vi "LIDAR 5.1 Unified Version V1.vi"() -> ()   [LabVIEW 2015]
uses:
  Controls/FPGA Nain State.ctl
  Controls/AI Slave State.ctl
  <vilib>/Platform/TimedLoop/XDataNode/timing_clust.ctl
  <vilib>/Platform/TimedLoop/XDataNode/nitl_modes.ctl
  <vilib>/Platform/TimedLoop/XDataNode/wakeup.ctl
  <vilib>/rvi/Emulation/niFpgaGetClockAttributes.vi
  <vilib>/rvi/Emulation/niFpgaSctlEmulationGetInTimedLoop.vi
  <vilib>/rvi/Emulation/niFpgaEmulationReportErrorSimple.vi
  <vilib>/rvi/eio/common/nirviEmuTemplateMethod_errors.vi
  <vilib>/rvi/Emulation/niFpgaCriticalErrorInLSC.vi
  LIDAR Slave Globals.vi
  <vilib>/rvi/Emulation/niFpgaProcessEmulError.vi
  <vilib>/rvi/Memory/Memory_Emulation/nirvimemoryFastEmulation.vi
  <vilib>/rvi/Memory/Memory_Emulation/nirvimemoryEmulation.vi
  <vilib>/rvi/Emulation/niFpgaEmulationIsFPGAContextNoSignature.vi
  <vilib>/rvi/DataTransferAndStorage/Container/Common/niFpgaContainerGetUniqueNameForEmu.vi
  <vilib>/rvi/errors/nirviReportUnexpectedCaseInternalError (U32).vi
  <vilib>/rvi/errors/niFpgaSetErrorForExecOnDevCompSimple.vi
  <vilib>/rvi/eio/common/nirviEmuReportErrorAndStop.vi
  <vilib>/rvi/FIFO/Fifo_Resource/nirvififoEmulationSetSize.vi
  <vilib>/rvi/FIFO/Fifo_Resource/nirviFifoEmulationQueueMgr.vi
  <instcachedir>/0/nirviFifoEmulationQueueMgr_E5CAEC123FF24DC58D834DCA3CDAA9B5.lvgen/nirviFifoEmulationQueueMgr_E5CAEC123FF24DC58D834DCA3CDAA9B5_003.vi
  <vilib>/Utility/error.llb/Clear Errors.vi
  <vilib>/rvi/FIFO/Fifo_Resource/nirvififoEmulationCreateLock.vi
  <vilib>/rvi/FIFO/Fifo_Resource/nirvififoEmulationObtainLock.vi
  <vilib>/rvi/FIFO/Fifo_Resource/nirvififoEmulationReleaseLock.vi
  <vilib>/rvi/occurrence/nirviWaitOnOccurrenceBase.vi
  <vilib>/rvi/errors/nirviReportUnexpectedCaseInternalError.vi
  <instcachedir>/0/nirviFifoEmulationQueueMgr_E5CAEC123FF24DC58D834DCA3CDAA9B5.lvgen/nirviFifoEmulationQueueMgr_E5CAEC123FF24DC58D834DCA3CDAA9B5_001.vi
  <vilib>/rvi/FIFO/Fifo_Resource/nirvififoEmulationDetermineInputValidOut.vi
  <vilib>/rvi/interface/RandomDataEmulation/niFpgaRandomDataHandleErrors.vi
  <vilib>/eio/EIONode/EIONode.xnode
  <vilib>/Platform/TimedLoop/XDataNode/XDataNode.xnode
  <vilib>/rvi/DataTransferAndStorage/Container/XNode/niFpgaContainer.xnode
  <vilib>/rvi/FIFO/Fifo_Resource/nirvififoEmulationRead.vi
  <vilib>/eio/EIOMethodNode/EIOMethodNode.xnode
  <vilib>/rvi/FIFO/Fifo_Resource/nirvififoEmulationWrite.vi
  <vilib>/rvi/interface/RandomDataEmulation/nirviRandomDataFpgaReadWriteTemplate.vi
  <vilib>/Platform/TimedLoop/XDataNode/XDNodeRunTimeDep.lvlib
  LIDAR V2 Globals.vi
panel:
  in  "Mode":bool
  in  "ResetTimeout":bool
  out "DMATimeout":bool
  in  "DebugValues":bool
  in  "TrigTimeout":u32=10000
  in  "OverrideTrig":bool
  out "SimSensID":u8
  out "FirstIterration":bool
  out "SamplesAmpount":u8
  out "VCSL#":u8
  out "AI Slave State":T1=enum."Error"
  in  "WriteSensAdd":i16
  in  "WriteSenseData":i16
  in  "WriteSensDataEn":bool
  out "User Command Idle":bool
  out "User Command Status":u8
  out "User Error":bool
  out "Configured?":bool
  out "PLL Locked":bool
  in  "User Data 0":u8
  in  "User Data 1":u8
  in  "User Command":u8
  in  "User Command Commit":bool
  in  "VgaAdd":u32
  in  "VgaData":i16
  in  "FillVga":bool
  in  "PowerBit0":bool
  in  "PowerBit1":bool
  in  "ActiveLedIndexDeb":u16
  in  "LedScanDebEn":bool
  out "Port0":u8=2 format="%.0b"
  out "Port1Bit4":bool
  out "Port1Bit5":bool
  out "Port1":u8 format="%.0b"
  in  "ScanMode":bool
  out "PulseIndex":i16=88
  in  "StartAcq":u16=26
  in  "StartPulse":u16=20
  in  "StartES":u16=15
  in  "StopES":u16=30
  out "EnableSignal":bool
  in  "PulseEnd":u16=25
  in  "DOActivate":u16=10
  in  "SendAiCMD":u16
  in  "NoOfSamples":u16=1247
  in  "AiNoOfSamples":u16
  in  "SensorMap":u8[](array[numeric])=[0, 0, 0, 0, 0, 0, 0, 0, 0, 0, 0, 0, 1, 1, 1, 1, 1, 1, 1, 1, 1, 1, 1, 1, 0, 0, 0, 0, 0, 0, 0, 0, 0, 0, 0, 0, 1, 1, 1, 1, 1, 1, 1, 1, 1, 1, 1, 1, 2, 2, 2, 2, 2, 2, 2, 2, 2, 2, 2, 2, 3, 3, 3, 3, 3, 3, 3, 3, 3, 3, 3, 3, 2, 2, 2, 2, 2, 2, 2, 2, 2, 2, 2, 2, 3, 3, 3, 3, 3, 3, 3, 3, 3, 3, 3, 3]
  in  "ActiveSensDeb":u8
  in  "SensScanDeb":bool
  in  "SendDebugVal":bool
  in  "EndOfPulseGen":bool=TRUE
  in  "SamplingEnable":bool
  in  "SingleFrame":bool
  out "MainState":T2=enum."ActivatePulseCycle"
  in  "NoOfLeds":u16=95
  in  "PulsePerLed":i16=199
  out "ActiveLedIndex":u16=2
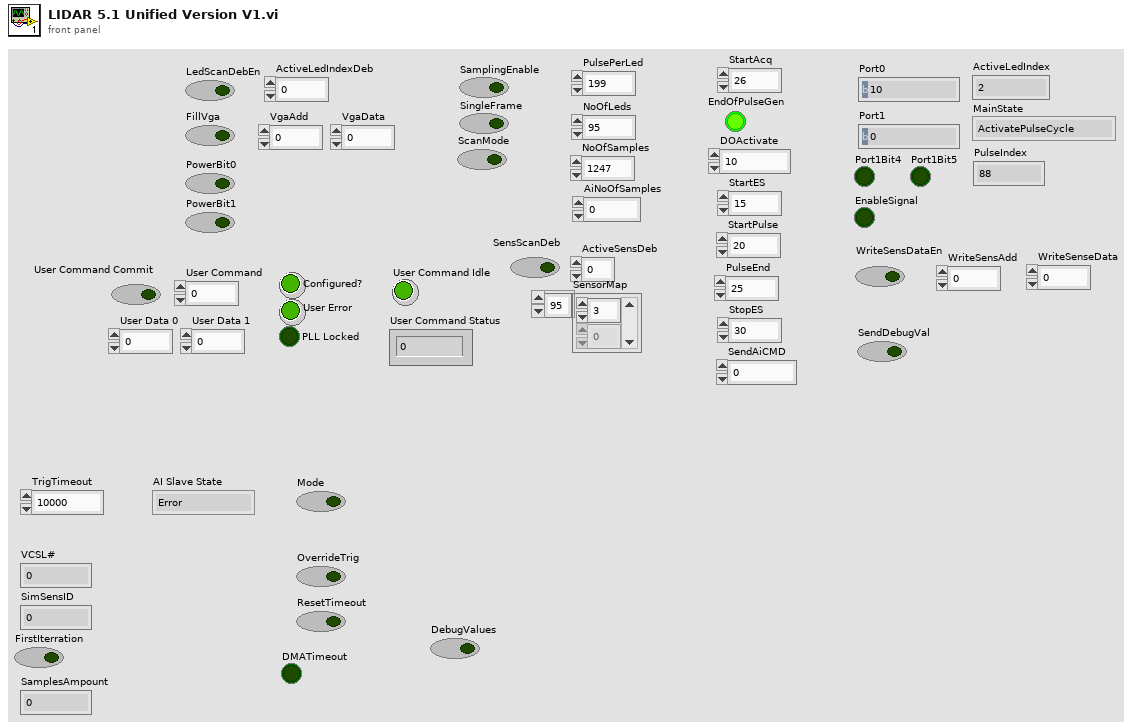
[diagram p1: front panel]
types:
  T1 = typedef "AI Slave State.ctl" = enum8{"WaitForStart", "WaitForTrig", "Read AI", "Error"}
  T2 = typedef "FPGA Nain State.ctl" = enum16{"WaitForStart", "SelectActiveLed", "WaitForNextPulse", "ActivatePulseCycle", "Error"}
  T3 = typedef "XDNodeRunTimeDep.lvlib/timing_clust.ctl" = cluster{"Expected End [f-1]":u64, "Actual End [f-1]":u64, "Finished Late? [f-1]":bool, "Expected End [i-1]":u64, "Actual End [i-1]":u64, "Finished Late? [i-1]":bool, "Expected Start [i]":u64, "Actual Start [i]":u64, "Expected Start [f]":u64, "Actual Start [f]":u64, "Source Name":string, "Structure Name":string, "Period":i64, "Deadline":i64, "Offset":i64, "Start":i64, "Priority":i32, "Timeout":i32, "Mode":T4, "Wakeup Reason":T5, "Error":errorcluster, "Source Type":string, "Secondary Source Type":string, "Global End Time":u64, "Global Start Time":u64, "Frame Duration":u64, "Iteration Duration":u64, "Assigned CPU":i32, "I/O Scan Engine Mode":u32}
  T4 = typedef "XDNodeRunTimeDep.lvlib/nitl_modes.ctl" = enum32{"No Change", "Process missed periods, maintain original phase", "Discard missed periods, maintain original phase", "Process missed periods, ignore original phase", "Discard missed periods, ignore original phase"}
  T5 = typedef "XDNodeRunTimeDep.lvlib/wakeup.ctl" = enum32{"Normal", "Aborted", "Asynchronous wakeup", "Timing source error", "Timed loop error", "Timeout"}
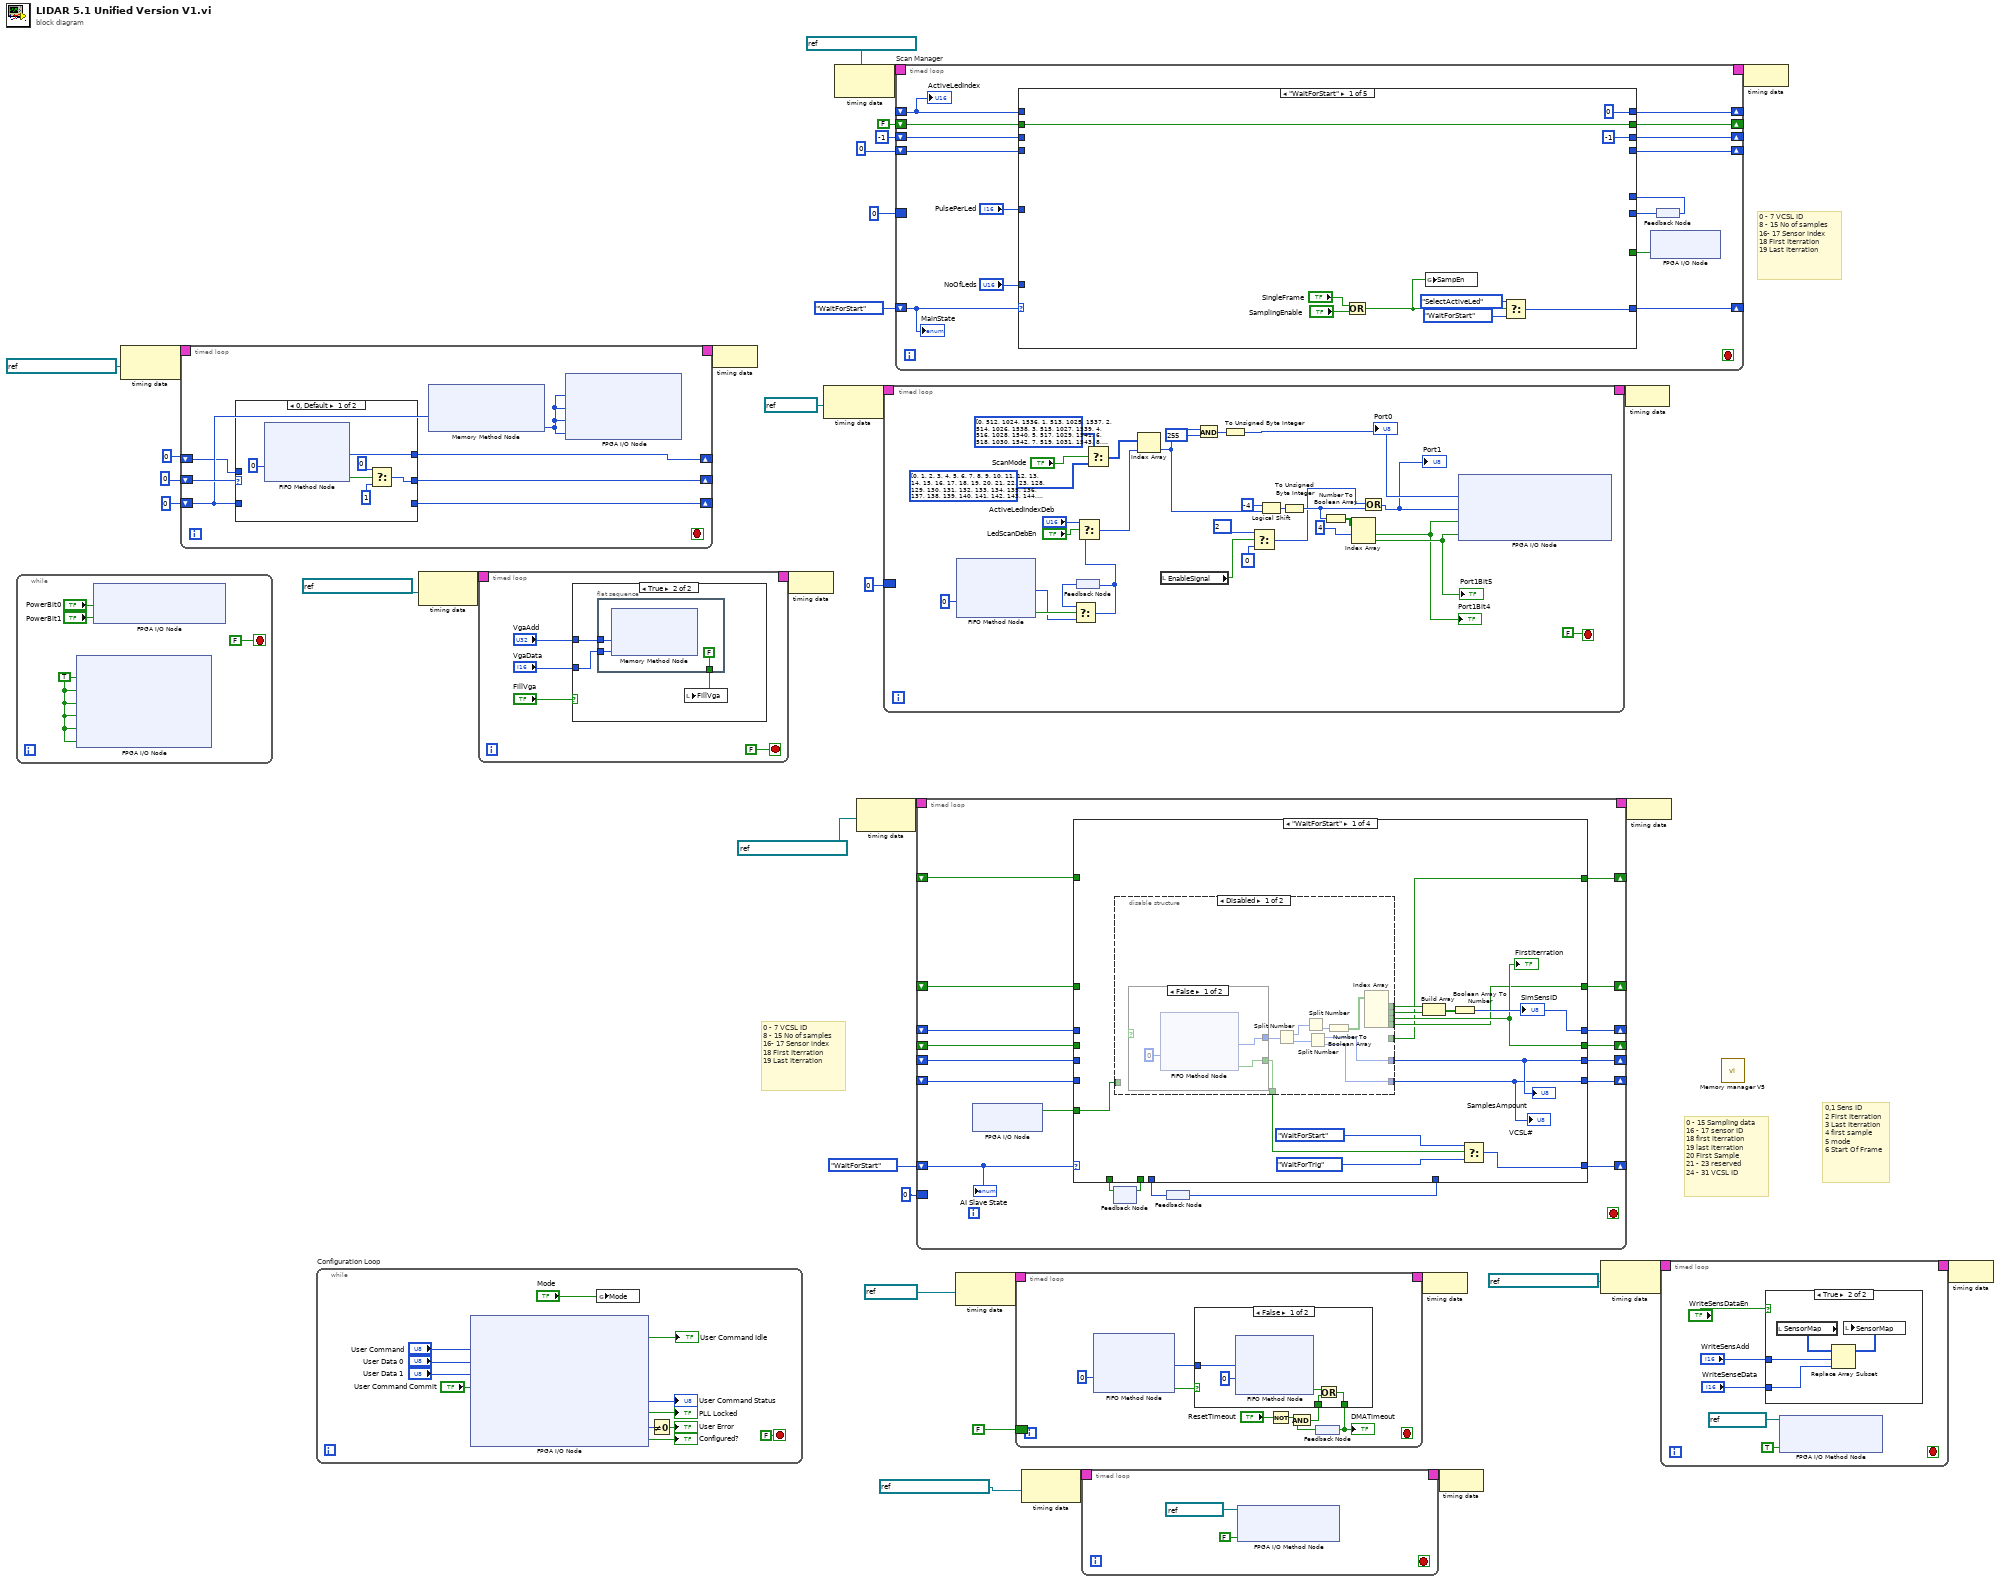
[diagram p0: block diagram]
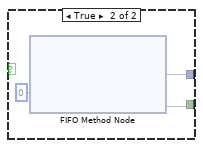
[diagram p3: hidden frame]
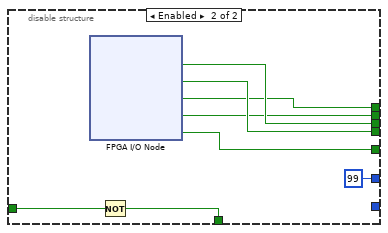
[diagram p4: hidden frame]
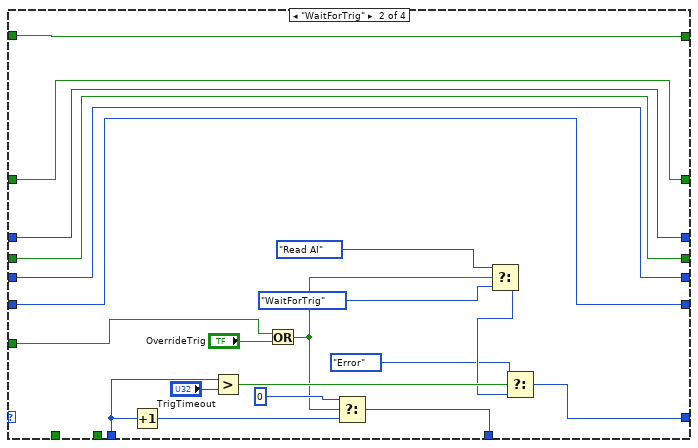
[diagram p5: hidden frame]
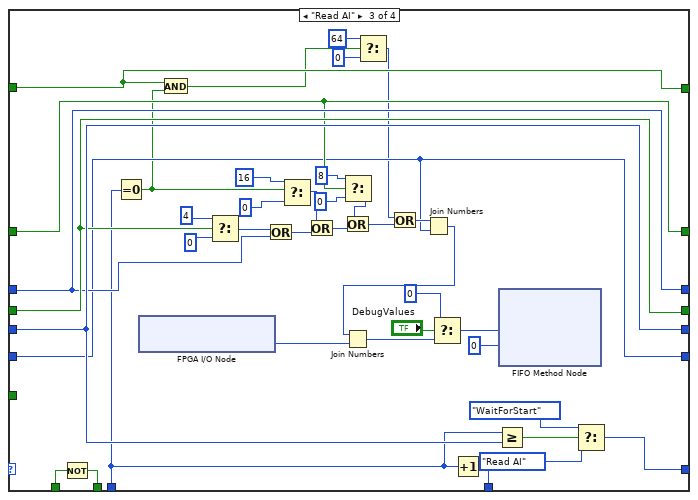
[diagram p6: hidden frame]
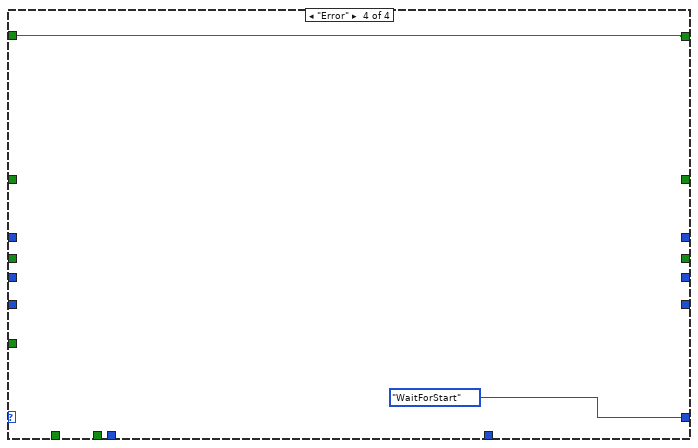
[diagram p7: hidden frame]
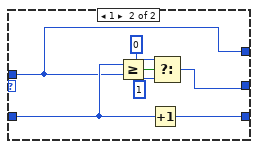
[diagram p9: hidden frame]
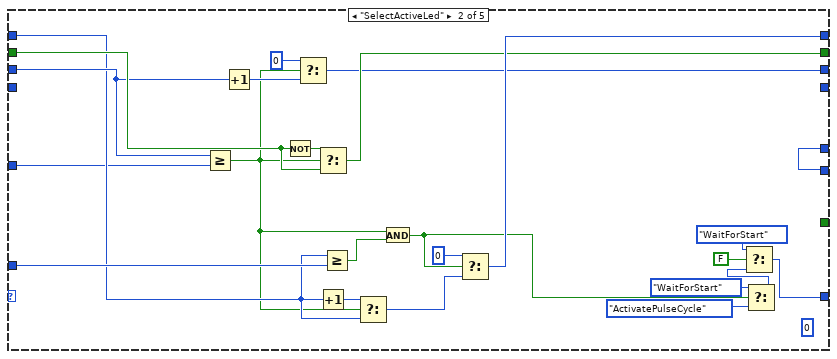
[diagram p11: hidden frame]
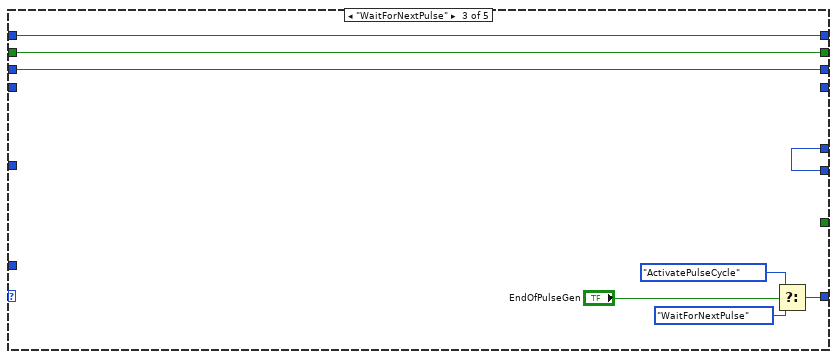
[diagram p12: hidden frame]
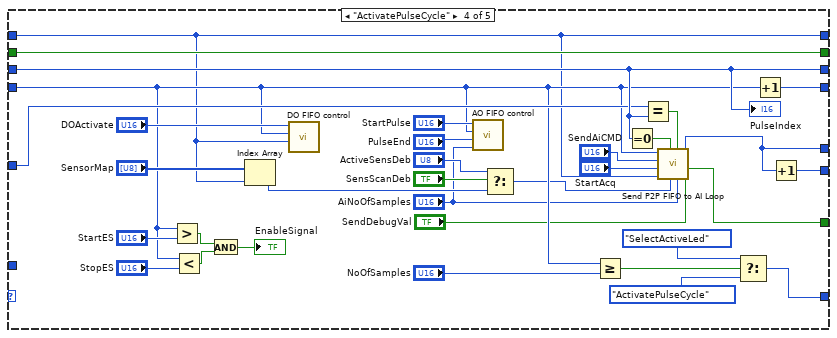
[diagram p13: hidden frame]
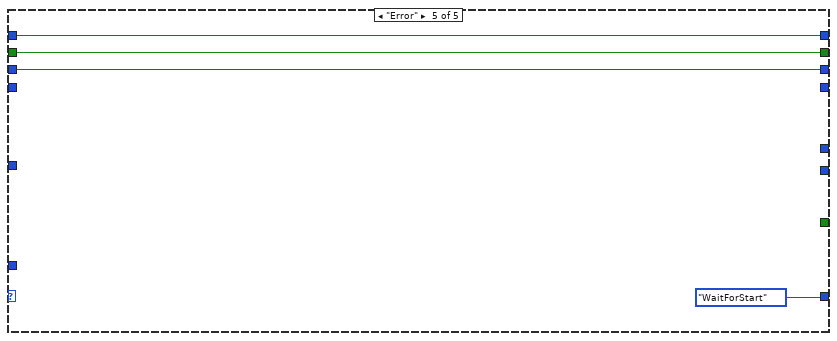
[diagram p14: hidden frame]
diagram:
  # "0,1 Sens ID\n2 First Iterration\n3 Last Iterration\n4 first sample\n5 mode\n6 Start Of Frame"
  # "0 - 15 Sampling data\n16 - 17 sensor ID\n18 first iterration\n19 last iterration\n20 First Sample\n21 - 23 reserved\n24 - 31 VCSL ID"
  # "0 - 7 VCSL ID\n8 - 15 No of samples\n16- 17 Sensor index\n18 First Iterration\n19 Last Iterration"
  # "0 - 7 VCSL ID\n8 - 15 No of samples\n16- 17 Sensor index\n18 First Iterration\n19 Last Iterration"
  n1 = while {
    stop <- FALSE stop-if-true
    w37 = TRUE ("IO Module\\PFI 0 WE")
    n2 = xnode "FPGA I/O Node"("IO Module\\PFI 0 WE"=w37, "IO Module\\PFI 1 WE"=w37, "IO Module\\PFI 2 WE"=w37, "IO Module\\PFI 3 WE"=w37, "IO Module\\DIO Port 0 WE"=w37, "IO Module\\DIO Port 1 WE"=w37) -> ()  [unwired: 6 in, 6 out]
    n3 = xnode "FPGA I/O Node"("IO Module\\PFI 2 Wr Data"="PowerBit0", "IO Module\\PFI 3 Wr Data"="PowerBit1") -> ()  [unwired: 2 in, 2 out]
  }
  n4 = node-c288(refnum<k21> "IO Module\\Data Clock" ("Source Name")) -> (w30:T3)
  n5 = timed-loop {
    timing: w30 -> [_]
    timing-out: [_] -> w29
    shift-right: [w44] -> _
    shift-left: u16 0 -> [w43]
    shift-right: [w45] -> _
    shift-left: u8 0 -> [w46]
    shift-right: [w42] -> _
    shift-left: u16 0 ("Element") -> [w41]
    stop <- _ stop-if-true
    n6 = case shown="0, Default" w46 {
      tunnel: [w49 w55] -> w45
      tunnel: w43 -> [_ w58]
      tunnel: [_ w60] -> w44
      tunnel: w41 -> [_ w54]
      tunnel: [w48 w54] -> w42
      frame 0, Default {
        n7 = xnode ("FIFO Method Node")("Timeout"=0) -> ("Element"=w48:u16, "Timed Out?"=w52:bool)  [unwired: 1 in, 1 out]
        n8 = Select(t=u8 0, s=w52, f=u8 1) -> (s? t:f=w49:u8)
      }
      frame 1 {
        n9 = Greater Or Equal?(x=w58, y=w54) -> (x >= y?=w59:bool)
        n10 = Increment(x=w58) -> (x+1=w60:u16)
        n11 = Select(t=u8 0, s=w59, f=u8 1) -> (s? t:f=w55:u8)
      }
    }
    n12 = xnode ("Memory Method Node")("Address"=w43) -> ("Data"=w47:i16)  [unwired: 1 in, 1 out]
    n13 = xnode "FPGA I/O Node"("IO Module\\AO 1 N-3"=w47, "IO Module\\AO 1 N-2"=w47, "IO Module\\AO 1 N-1"=w47, "IO Module\\AO 1 N"=w47) -> ()  [unwired: 4 in, 4 out]
  }
  n14 = while "Configuration Loop" {
    stop <- FALSE stop-if-true
    n15 = xnode "FPGA I/O Node"("IO Module\\User Command"="User Command", "IO Module\\User Data 0"="User Data 0", "IO Module\\User Data 1"="User Data 1", "IO Module\\User Command Commit"="User Command Commit") -> ("IO Module\\User Command Idle"=→"User Command Idle":bool, "IO Module\\User Command Status"=→"User Command Status":u8, "IO Module\\PLL Locked"=→"PLL Locked":bool, "IO Module\\User Error"=w71:u8, "IO Module\\Initialization Done"=→"Configured?":bool)  [unwired: 9 in, 9 out]
    n16 = global write "LIDAR Slave Globals.vi" "Mode"("Mode") -> ()
    n17 = Not Equal To 0?(x=w71) -> (x != 0?=→"User Error":bool)
  }
  n18 = node-c288(refnum<k21> "IO Module\\Data Clock" ("Source Name")) -> (w32:T3)
  n19 = timed-loop {
    timing: w32 -> [_]
    timing-out: [_] -> w31
    stop <- FALSE stop-if-true
    n20 = case shown="True" "FillVga" {
      tunnel: "VgaAdd" -> [_ w81]
      tunnel: "VgaData" -> [_ w80]
      frame False {
      }
      frame True {
        n21 = flat-sequence {
          tunnel: w81 -> [w84]
          tunnel: w80 -> [w83]
          tunnel: [FALSE ("FillVga")] -> w79
          frame #0 {
            n22 = xnode ("Memory Method Node")("Address"=w84, "Data"=w83) -> ()  [unwired: 1 in, 1 out]
          }
        }
        n23 = local write "FillVga"(w79) -> ()
      }
    }
  }
  n24 = node-c288(w29) -> ()
  n25 = node-c288(w31) -> ()
  n26 = node-c288(refnum<k21> "130MHz" ("Source Name")) -> (w34:T3)
  n27 = node-c288(refnum<k21> "IO Module\\Data Clock" ("Source Name")) -> (w36:T3)
  n28 = node-c288(refnum<k21> "IO Module\\Data Clock" ("Source Name")) -> (w12:T3)
  n29 = timed-loop {
    timing: w34 -> [_]
    timing-out: [_] -> w33
    border: u16 0 ("Element") -> [_]
    stop <- FALSE stop-if-true
    n30 = xnode ("FIFO Method Node")("Timeout"=0) -> ("Element"=w95:u16, "Timed Out?"=w96:bool)  [unwired: 1 in, 1 out]
    n31 = feedback #1() -> (w93:u16)
    n32 = Select(t=w93, s=w96, f=w95) -> (s? t:f=w94:u16)
    n33 = feedback-in #1(w94) -> ()
    n34 = Select(t="ActiveLedIndexDeb", s="LedScanDebEn", f=w94) -> (s? t:f=w104:u16)
    n35 = Select(t=u16[] [0, 512, 1024, 1536, 1, 513, 1025, 1537, 2, 514, 1026, 1538, 3, 515, 1027, 1539, 4, 516, 1028, 1540, 5, 517, 1029, 1541, 6, 518, 1030, 1542, 7, 519, 1031, 1543, 8, 520, 1032, 1544, 9, 521, 1033, 1545, 10, 522, 1034, 1546, 11, 523, 1035, 1547, 12, 524, 1036, 1548, 13, 525, 1037, 1549, 14, 526, 1038, 1550, 15, 527, 1039, 1551, 16, 528, 1040, 1552, 17, 529, 1041, 1553, 18, 530, 1042, 1554, 19, 531, 1043, 1555, 20, 532, 1044, 1556, 21, 533, 1045, 1557, 22, 534, 1046, 1558, 23, 535, 1047, 1559, 0, 0, 0, 0, 0, 0, 0, 0, 0, 0, 0, 0, 0, 0, 0, 0, 0, 0, 0, 0, 0, 0, 0, 0, 0, 0, 0, 0, 0, 0, 0, 0, 0, 0, 0, 0, 0, 0, 0, 0, 0, 0, 0, 0, 0, 0, 0, 0, 0, 0, 0, 0, 0, 0, 0, 0, 0, 0, 0, 0, 0, 0, 0, 0, 0, 0, 0, 0, 0, 0, 0, 0, 0, 0, 0, 0, 0, 0, 0, 0, 0, 0, 0, 0, 0, 0, 0, 0, 0, 0, 0, 0, 0, 0, 0, 0, 0, 0, 0, 0, 0, 0, 0, 0, 0, 0, 0, 0, 0, 0, 0, 0, 0, 0, 0, 0, 0, 0, 0, 0, 0, 0, 0, 0, 0, 0, 0, 0, 0, 0, 0, 0, 0, 0, 0, 0, 0, 0, 0, 0, 0, 0, 0, 0, 0, 0, 0, 0, 0, 0, 0, 0, 0, 0, 0, 0, 0, 0, 0, 0, 0, 0, 0, 0, 0, 0, 0, 0, 0, 0, 0, 0, 0, 0, 0, 0, 0, 0, 0, 0, 0, 0, 0, 0, 0, 0, 0, 0, 0, 0, 0, 0, 0, 0, 0, 0, 0, 0, 0, 0, 0, 0, 0, 0, 0, 0, 0, 0, 0, 0, 0, 0, 0, 0, 0, 0, 0, 0, 0, 0, 0, 0, 0, 0] ("Array"), s="ScanMode", f=u16[] [0, 1, 2, 3, 4, 5, 6, 7, 8, 9, 10, 11, 12, 13, 14, 15, 16, 17, 18, 19, 20, 21, 22, 23, 128, 129, 130, 131, 132, 133, 134, 135, 136, 137, 138, 139, 140, 141, 142, 143, 144, 145, 146, 147, 148, 149, 150, 151, 256, 257, 258, 259, 260, 261, 262, 263, 264, 265, 266, 267, 268, 269, 270, 271, 272, 273, 274, 275, 276, 277, 278, 279, 384, 385, 386, 387, 388, 389, 390, 391, 392, 393, 394, 395, 396, 397, 398, 399, 400, 401, 402, 403, 404, 405, 406, 407, 0, 0, 0, 0, 0, 0, 0, 0, 0, 0, 0, 0, 0, 0, 0, 0, 0, 0, 0, 0, 0, 0, 0, 0, 0, 0, 0, 0, 0, 0, 0, 0, 0, 0, 0, 0, 0, 0, 0, 0, 0, 0, 0, 0, 0, 0, 0, 0, 0, 0, 0, 0, 0, 0, 0, 0, 0, 0, 0, 0, 0, 0, 0, 0, 0, 0, 0, 0, 0, 0, 0, 0, 0, 0, 0, 0, 0, 0, 0, 0, 0, 0, 0, 0, 0, 0, 0, 0, 0, 0, 0, 0, 0, 0, 0, 0, 0, 0, 0, 0, 0, 0, 0, 0, 0, 0, 0, 0, 0, 0, 0, 0, 0, 0, 0, 0, 0, 0, 0, 0, 0, 0, 0, 0, 0, 0, 0, 0, 0, 0, 0, 0, 0, 0, 0, 0, 0, 0, 0, 0, 0, 0, 0, 0, 0, 0, 0, 0, 0, 0, 0, 0, 0, 0, 0, 0, 0, 0, 0, 0, 0, 0, 0, 0, 0, 0, 0, 0, 0, 0, 0, 0, 0, 0, 0, 0, 0, 0, 0, 0, 0, 0, 0, 0, 0, 0, 0, 0, 0, 0, 0, 0, 0, 0, 0, 0, 0, 0, 0, 0, 0, 0, 0, 0, 0, 0, 0, 0, 0, 0, 0, 0, 0, 0, 0, 0, 0, 0, 0, 0, 0, 0, 0, 0] ("Array")) -> (s? t:f=w99:u16[])
    n36 = Index Array(array=w99, index=w104) -> (element=w89:u16)
    n37 = local read "EnableSignal"() -> (w97:bool)
    n38 = And(x=w89, y=u16 255) -> (x .and. y?=w109:u16)
    n39 = To Unsigned Byte Integer(number=w109) -> (unsigned 8bit integer=w107:u8)
    "Port0" <- w107
    n40 = Select(t=u8 2, s=w97, f=u8 0) -> (s? t:f=w88:u8)
    n41 = Logical Shift(y=i16 -4, x=w89) -> (x << y=w108:u16)
    n42 = To Unsigned Byte Integer(number=w108) -> (unsigned 8bit integer=w106:u8)
    n43 = Number To Boolean Array(number=w106) -> (Boolean array=w113:bool[])
    n44 = Index Array(array=w113, index #1=4 ("index")) -> (element #1=w91:bool, element #2=w92:bool)  [unwired: 1 in]
    "Port1Bit4" <- w91
    "Port1Bit5" <- w92
    n45 = Or(x=w88, y=w106) -> (x .or. y?=w105:u8)
    "Port1" <- w105
    n46 = xnode "FPGA I/O Node"("IO Module\\DIO Port 0 Wr Data"=w107, "IO Module\\DIO Port 1 Wr Data"=w105, "IO Module\\PFI 0 Wr Data"=w91, "IO Module\\PFI 1 Wr Data"=w92) -> ()  [unwired: 4 in, 4 out]
  }
  n47 = timed-loop "Scan Manager" {
    timing: w36 -> [_]
    timing-out: [_] -> w35
    shift-right: [w131] -> _
    shift-left: FPGA_Nain_State."WaitForStart" ("MainState") -> [w132]
    shift-right: [w126] -> _
    shift-left: _ -> [w121]
    shift-right: [w128] -> _
    shift-left: FALSE -> [w130]
    shift-right: [w129] -> _
    shift-left: i16 -1 -> [w127]
    shift-right: [w122] -> _
    shift-left: u16 0 -> [w123]
    border: u32 0 -> [_]
    stop <- _ stop-if-true
    n48 = feedback #2() -> (w118:u32)
    n49 = case shown="\"WaitForStart\"" w132 {
      tunnel: [w139 w162 w169 w203 FPGA_Nain_State."WaitForStart" ("MainState")] -> w131
      tunnel: [u16 0 ("ActiveLedIndex") w158 w168 w182 w210] -> w126
      tunnel: w121 -> [_ w150 w168 w182 w210]
      tunnel: [w136 w157 w173 w202 w209] -> w128
      tunnel: w130 -> [w136 w160 w173 w202 w209]
      tunnel: [i16 -1 ("t") w153 w172 w187 w208] -> w129
      tunnel: w127 -> [_ w156 w172 w187 w208]
      tunnel: "NoOfLeds" -> [_ w152 _ _ _]
      tunnel: "PulsePerLed" -> [_ w143 _ w186 _]
      tunnel: w123 -> [_ _ _ w183 _]
      tunnel: [_ _ _ w201 _] -> w122
      tunnel: [_ _ _ w178 _] -> w120
      tunnel: w118 -> [_ w142 w166 w176 _]
      tunnel: [_ w142 w166 w177 _] -> w119
      frame "WaitForStart" {
        n50 = Or(x="SingleFrame", y="SamplingEnable") -> (x .or. y?=w133:bool)
        n51 = global write "LIDAR V2 Globals.vi" "SampEn"(w133) -> ()
        n52 = Select(t=FPGA_Nain_State."SelectActiveLed" ("MainState"), s=w133, f=FPGA_Nain_State."WaitForStart" ("MainState")) -> (s? t:f=w139:T2)
      }
      frame "SelectActiveLed" {
        (unwired) u8 0
        n53 = Greater Or Equal?(x=w156, y=w143) -> (x >= y?=w145:bool)
        n54 = Increment(x=w156) -> (x+1=w155:i16)
        n55 = Not(x=w160) -> (.not. x?=w159:bool)
        n56 = Select(t=i16 0, s=w145, f=w155) -> (s? t:f=w153:i16)
        n57 = Select(t=w159, s=w145, f=w160) -> (s? t:f=w157:bool)
        n58 = Increment(x=w150) -> (x+1=w148:u16)
        n59 = Greater Or Equal?(x=w150, y=w152) -> (x >= y?=w146:bool)
        n60 = Select(t=w148, s=w145, f=w150) -> (s? t:f=w149:u16)
        n61 = And(x=w145, y=w146) -> (x .and. y?=w144:bool)
        n62 = Select(t=u16 0, s=w144, f=w149) -> (s? t:f=w158:u16)
        n63 = Select(t=FPGA_Nain_State."WaitForStart" ("MainState"), s=w144, f=FPGA_Nain_State."ActivatePulseCycle" ("MainState")) -> (s? t:f=w163:T2)
        n64 = Select(t=FPGA_Nain_State."WaitForStart" ("MainState"), s=FALSE, f=w163) -> (s? t:f=w162:T2)
      }
      frame "WaitForNextPulse" {
        n65 = Select(t=FPGA_Nain_State."ActivatePulseCycle" ("MainState"), s="EndOfPulseGen", f=FPGA_Nain_State."WaitForNextPulse" ("MainState")) -> (s? t:f=w169:T2)
      }
      frame "ActivatePulseCycle" {
        n66 = Greater?(x=w183, y="StartES") -> (0:w196:bool)
        n67 = Less?(x=w183, y="StopES") -> (x < y?=w197:bool)
        n68 = And(x=w196, y=w197) -> (x .and. y?=→"EnableSignal":bool)
        n69 = Index Array(array="SensorMap", index=w182) -> (element=w181:u8)
        n70 = call "DO FIFO control.vi"("PulseData"=w182, "Counter"=w183, "DOActivate"="DOActivate") -> ()  [unwired: 9 in]
        n71 = call "AO FIFO control.vi"("NoOfSamples"="AiNoOfSamples", "PulseEnd"="PulseEnd", "Counter"=w183, "PulseStart"="StartPulse") -> ()  [unwired: 8 in]
        n72 = Select(t="ActiveSensDeb", s="SensScanDeb", f=w181) -> (s? t:f=w180:u8)
        n73 = Greater Or Equal?(x=w183, y="NoOfSamples") -> (x >= y?=w206:bool)
        n74 = Equal To 0?(x=w187) -> (x = 0?=w189:bool)
        n75 = Equal?(x=w186, y=w187) -> (x = y?=w188:bool)
        n76 = call "Send P2P FIFO to AI Loop.vi"("SendDebugVal"="SendDebugVal", "DebugVals"=w176, "NoOfSamples"="AiNoOfSamples", "LastIterration"=w188, "SensorID"=w180, "FirstIterration"=w189, "ActiveLedIndex"=w182, "SendAiTrig"="StartAcq", "SendAiCMD"="SendAiCMD", "TimingCounter"=w183) -> ("Trig"=w178:bool)  [unwired: 1 out]
        n77 = Select(t=FPGA_Nain_State."SelectActiveLed" ("MainState"), s=w206, f=FPGA_Nain_State."ActivatePulseCycle" ("MainState")) -> (s? t:f=w203:T2)
        n78 = Increment(x=w183) -> (x+1=w201:u16)
        n79 = Increment(x=w176) -> (x+1=w177:u32)
        "PulseIndex" <- w187
      }
      frame "Error" {
      }
    }
    n80 = xnode "FPGA I/O Node"("PXI_Trig0"=w120) -> ()  [unwired: 1 in, 1 out]
    n81 = feedback-in #2(w119) -> ()
    "MainState" <- w132
    "ActiveLedIndex" <- w121
  }
  n82 = timed-loop {
    timing: w12 -> [_]
    timing-out: [_] -> w11
    shift-right: [w231] -> _
    shift-left: AI_Slave_State."WaitForStart" -> [w220]
    shift-right: [w230] -> _
    shift-left: _ -> [w229]
    shift-right: [w228] -> _
    shift-left: _ -> [w227]
    shift-right: [w226] -> _
    shift-left: _ -> [w225]
    shift-right: [w224] -> _
    shift-left: _ -> [w223]
    border: i16 0 -> [_]
    shift-right: [w219] -> _
    shift-left: _ -> [w218]
    shift-right: [w214] -> _
    shift-left: _ -> [w213]
    stop <- _ stop-if-true
    n83 = xnode "FPGA I/O Node"() -> ("PXI_Trig0"=w217:bool)  [unwired: 1 in, 1 out]
    n84 = feedback #3() -> (w216:bool)  [unwired: 1 in]
    n85 = feedback #4() -> (w222:i16)
    n86 = case shown="\"WaitForStart\"" w220 {
      tunnel: [w242 w280 w324 AI_Slave_State."WaitForStart"] -> w231
      tunnel: [w238 w288 w301 _] -> w230
      tunnel: w229 -> [_ w288 w301 _]
      tunnel: [w239 w289 w328 _] -> w228
      tunnel: w227 -> [_ w289 w328 _]
      tunnel: [w240 w290 w323 _] -> w226
      tunnel: w225 -> [_ w290 w323 _]
      tunnel: [w241 w291 w320 _] -> w224
      tunnel: w223 -> [_ w291 w320 _]
      tunnel: w222 -> [_ w285 w307 _]
      tunnel: [_ w278 w329 _] -> w221
      tunnel: w217 -> [w233 w274 _ _]
      tunnel: [w234 w273 w309 _] -> w219
      tunnel: w218 -> [_ w273 w309 _]
      tunnel: [_ _ w306 _] -> w215
      tunnel: w216 -> [_ _ w305 _]
      tunnel: [w232 w272 w299 w331] -> w214
      tunnel: w213 -> [_ w272 w299 w331]
      frame "WaitForStart" {
        n87 = disable-structure shown="Disabled" {
          disable-tunnel: [w257 w266] -> w245
          disable-tunnel: [w256 w271] -> w240
          disable-tunnel: [w255 u8 99 ("SamplesAmpount")] -> w239
          disable-tunnel: [w254 _] -> w238
          disable-tunnel: [w248 w269] -> w237
          disable-tunnel: [w247 w268] -> w236
          disable-tunnel: [w246 w270] -> w234
          disable-tunnel: w233 -> [_ w267]
          disable-tunnel: [_ w264] -> w232
          frame Disabled {
            n88 = case shown="False" {
              selector: _ -> [_ _]
              tunnel: [w259 w261] -> w257
              tunnel: [w260 w262] -> w253
              frame False {
                n89 = xnode ("FIFO Method Node")("Timeout"=0) -> ("Element"=w260:u32, "Timed Out?"=w259:bool)  [unwired: 1 in, 1 out]
              }
              frame True {
                n90 = xnode ("FIFO Method Node")("Timeout"=0) -> ("Element"=w262, "Timed Out?"=w261)  [unwired: 1 in, 1 out]
              }
            }
            n91 = Split Number(x=w253) -> (hi(x)=w251:u16, lo(x)=w252:u16)
            n92 = Split Number(x=w251) -> (lo(x)=w250:u8)  [unwired: 1 out]
            n93 = Split Number(x=w252) -> (hi(x)=w255:u8, lo(x)=w254:u8)
            n94 = Number To Boolean Array(number=w250) -> (Boolean array=w249:bool[])
            n95 = Index Array(array=w249) -> (element #1=w248:bool, element #2=w247:bool, element #3=w256:bool, element #4=w246:bool)  [unwired: 4 in]
          }
          frame Enabled {
            n96 = xnode "FPGA I/O Node"() -> ("PXI_Trig2"=w271:bool, "PXI_Trig3"=w270:bool, "PXI_Trig4"=w269:bool, "PXI_Trig5"=w268:bool, "PXI_Trig6"=w264:bool)  [unwired: 5 in, 5 out]
            n97 = Not(x=w267) -> (.not. x?=w266:bool)
          }
        }
        "FirstIterration" <- w240
        "SamplesAmpount" <- w239
        "VCSL#" <- w238
        n98 = Build Array(w237, w236) -> (w235:bool[])
        n99 = Boolean Array To Number(Boolean array=w235) -> (number=w241:u8)
        "SimSensID" <- w241
        n100 = Select(t=AI_Slave_State."WaitForStart", s=w245, f=AI_Slave_State."WaitForTrig") -> (s? t:f=w242:T1)
      }
      frame "WaitForTrig" {
        n101 = Increment(x=w285) -> (x+1=w279:i16)
        n102 = Greater?(x=w285, y="TrigTimeout") -> (0:w283:bool)
        n103 = Or(x=w274, y="OverrideTrig") -> (x .or. y?=w276:bool)
        n104 = Select(t=i16 0, s=w276, f=w279) -> (s? t:f=w278:i16)
        n105 = Select(t=AI_Slave_State."Read AI", s=w276, f=AI_Slave_State."WaitForTrig") -> (s? t:f=w282:T1)
        n106 = Select(t=AI_Slave_State."Error", s=w283, f=w282) -> (s? t:f=w280:T1)
      }
      frame "Read AI" {
        n107 = Not(x=w305) -> (.not. x?=w306:bool)
        n108 = Equal To 0?(x=w307) -> (x = 0?=w300:bool)
        n109 = xnode "FPGA I/O Node"() -> ("IO Module\\AI 0 N"=w295:i16)  [unwired: 1 in, 1 out]
        n110 = And(x=w299, y=w300) -> (x .and. y?=w298:bool)
        n111 = Select(t=u8 4, s=w323, f=u8 0) -> (s? t:f=w321:u8)
        n112 = Or(x=w321, y=w320) -> (x .or. y?=w317:u8)
        n113 = Select(t=u8 16, s=w300, f=u8 0) -> (s? t:f=w314:u8)
        n114 = Or(x=w314, y=w317) -> (x .or. y?=w312:u8)
        n115 = Select(t=u8 8, s=w309, f=u8 0) -> (s? t:f=w308:u8)
        n116 = Or(x=w308, y=w312) -> (x .or. y?=w296:u8)
        n117 = Select(t=u8 64, s=w298, f=u8 0) -> (s? t:f=w297:u8)
        n118 = Or(x=w297, y=w296) -> (x .or. y?=w302:u8)
        n119 = Join Numbers(hi=w302, lo=w301) -> ((hi.lo)=w319:u16)
        n120 = Join Numbers(hi=w319, lo=w295) -> ((hi.lo)=w294:u32)
        n121 = Select(t=u32 0, s="DebugValues", f=w294) -> (s? t:f=w293:u32)
        n122 = Increment(x=w307) -> (x+1=w329:i16)
        n123 = Greater Or Equal?(x=w307, y=w328) -> (x >= y?=w327:bool)
        n124 = xnode ("FIFO Method Node")("Element"=w293, "Timeout"=0) -> ()  [unwired: 1 in, 2 out]
        n125 = Select(t=AI_Slave_State."WaitForStart", s=w327, f=AI_Slave_State."Read AI") -> (s? t:f=w324:T1)
      }
      frame "Error" {
      }
    }
    n126 = feedback-in #3(w215) -> ()
    n127 = feedback-in #4(w221) -> ()
    "AI Slave State" <- w220
  }
  n128 = node-c288(refnum<k21> "130MHz" ("Source Name")) -> (w10:T3)
  n129 = timed-loop {
    timing: w10 -> [_]
    timing-out: [_] -> w9
    border: FALSE -> [_]
    stop <- _ stop-if-true
    n130 = xnode ("FIFO Method Node")("Timeout"=0) -> ("Element"=w340:u32, "Timed Out?"=w342:bool)  [unwired: 1 in, 1 out]
    n131 = Not(x="ResetTimeout") -> (.not. x?=w335:bool)
    n132 = feedback #5() -> (w337:bool)
    n133 = And(x=w335, y=w337) -> (x .and. y?=w338:bool)
    n134 = case shown="False" w342 {
      tunnel: w340 -> [w347 _]
      tunnel: [w344 w348] -> w339
      tunnel: w338 -> [w343 w348]
      frame False {
        n135 = xnode ("FIFO Method Node")("Element"=w347, "Timeout"=0) -> ("Timed Out?"=w345:bool)  [unwired: 1 in, 1 out]
        n136 = Or(x=w345, y=w343) -> (x .or. y?=w344:bool)
      }
      frame True {
      }
    }
    "DMATimeout" <- w339
    n137 = feedback-in #5(w339) -> ()
  }
  n138 = node-c288(refnum<k21> "IO Module\\Data Clock" ("Source Name")) -> (w8:T3)
  n139 = timed-loop {
    timing: w8 -> [_]
    timing-out: [_] -> w7
    stop <- _ stop-if-true
    n140 = xnode "FPGA I/O Method Node"("FPGA I/O In"=refnum<k21> "PXI_Trig0", "Enable"=FALSE) -> ()  [unwired: 1 out]
  }
  n141 = node-c288(w9) -> ()
  n142 = node-c288(w7) -> ()
  n143 = node-c288(refnum<k21> "IO Module\\Data Clock" ("Source Name")) -> (w28:T3)
  n144 = node-c288(w33) -> ()
  n145 = node-c288(w11) -> ()
  n146 = timed-loop {
    timing: w28 -> [_]
    timing-out: [_] -> w27
    stop <- _ stop-if-true
    n147 = case shown="True" "WriteSensDataEn" {
      tunnel: "WriteSensAdd" -> [_ w361]
      tunnel: "WriteSenseData" -> [_ w360]
      frame False {
      }
      frame True {
        n148 = local read "SensorMap"() -> (w363:u8[])
        n149 = Replace Array Subset(array=w363, new element=w360, index=w361) -> (w362:u8[])
        n150 = local write "SensorMap"(w362) -> ()
      }
    }
    n151 = xnode "FPGA I/O Method Node"("FPGA I/O In"=refnum<k21> "PXI_Trig0", "Enable"=TRUE) -> ()  [unwired: 1 out]
  }
  n152 = call "Memory manager V5.vi"() -> ()  [unwired: 12 in]
  n153 = node-c288(w35) -> ()
  n154 = node-c288(w27) -> ()
